vi "Cook Dinner.vi"() -> ()   [LabVIEW 2011]
uses:
  Chef/Chef.lvclass
  Microwave/Microwave.lvclass
  Toaster/Toaster.lvclass
  Oven/Oven.lvclass
panel:
  in  "Steam":bool
  in  "Toast":bool
  in  "Stop":bool
  in  "Broil":bool
  in  "Braise":bool
  in  "Bake":bool
  in  "Select Appliance":string(combo)="Oven"
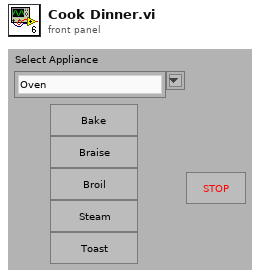
[diagram p1: front panel]
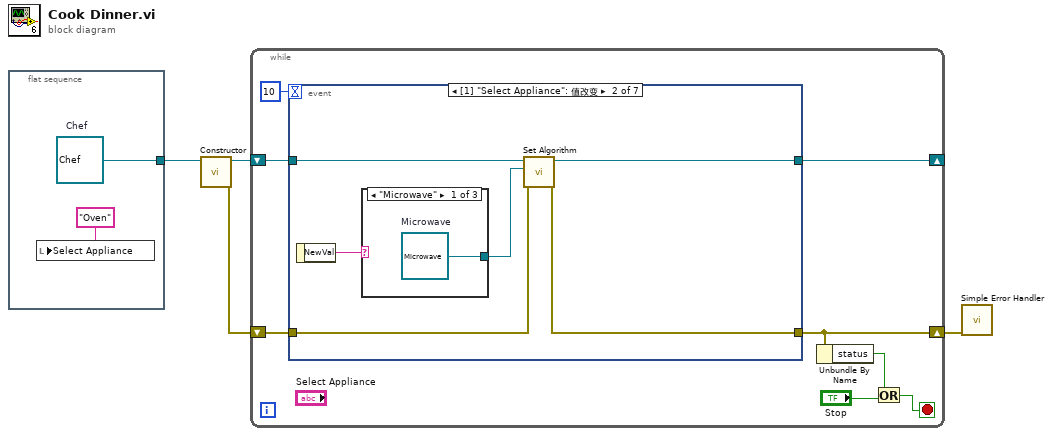
[diagram p0: block diagram]
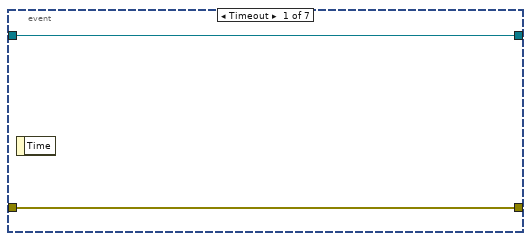
[diagram p2: hidden frame]
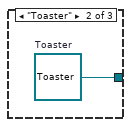
[diagram p3: hidden frame]
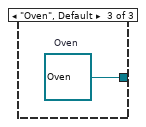
[diagram p4: hidden frame]
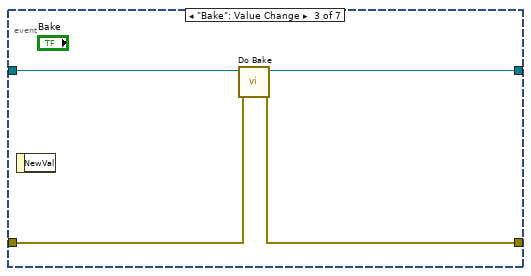
[diagram p5: hidden frame]
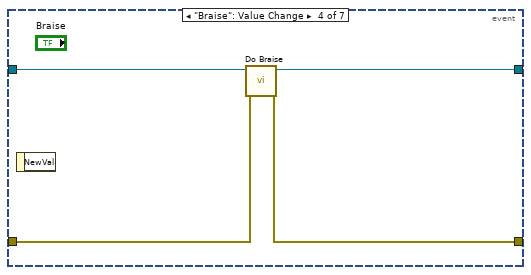
[diagram p6: hidden frame]
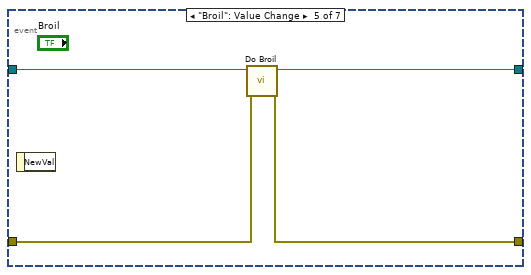
[diagram p7: hidden frame]
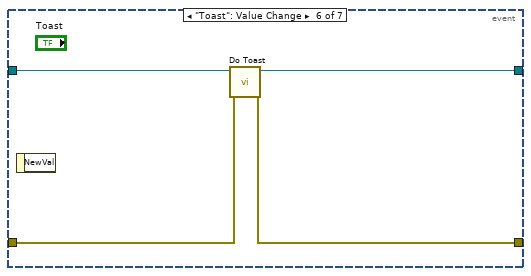
[diagram p8: hidden frame]
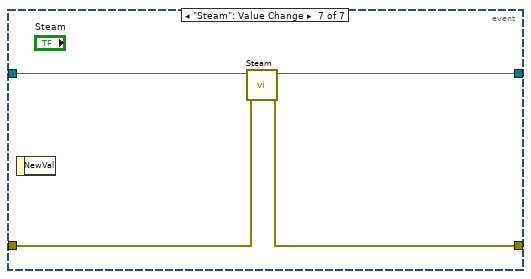
[diagram p9: hidden frame]
diagram:
  n1 = flat-sequence {
    tunnel: [w6] -> w4
    frame #0 {
      w6 = refnum<class "Chef.lvclass"> refnum  # Chef
      n2 = local write "Select Appliance"("Oven") -> ()
    }
  }
  n3 = call-dynamic "Constructor.vi"("Chef in"=w4) -> ("error out"=w2:errorcluster, "Chef out"=w3:refnum<class "Chef.lvclass">)  [unwired: 9 in]
  n4 = while {
    shift-right: [w12] -> _
    shift-left: w3 -> [w14]
    shift-right: [w11] -> w1
    shift-left: w2 -> [w13]
    stop <- w9 stop-if-true
    n5 = event shown="[1] \"Select Appliance\": 值改变" {
      selector: _ -> [_ _ _ _ _ _ _]
      dyn-events: _ -> [_ _ _ _ _ _ _]
      timeout: 10 -> [_ _ _ _ _ _ _]
      tunnel: w14 -> [w16 w22 w29 w33 w37 w41 w45]
      tunnel: [w15 w20 w26 w30 w34 w38 w42] -> w11
      tunnel: w13 -> [w15 w19 w27 w31 w35 w39 w43]
      tunnel: [w16 w18 w28 w32 w36 w40 w44] -> w12
      event Timeout {
        n6 = event-data() -> ()  [unwired: 1 in, 1 out]
      }
      event "Select Appliance": Value Change {
        n7 = event-data() -> ("NewVal"=w21:string)  [unwired: 1 in]
        n8 = case shown="\"Microwave\"" w21 {
          tunnel: [w23 w24 w25] -> w17
          frame "Microwave" {
            w23 = refnum<class "Microwave.lvclass"> refnum  # Microwave
          }
          frame "Toaster" {
            w24 = refnum<class "Toaster.lvclass"> refnum  # Toaster
          }
          frame "Oven", Default {
            w25 = refnum<class "Oven.lvclass"> refnum  # Oven
          }
        }
        n9 = call-dynamic "Set Algorithm.vi"("error in (no error)"=w19, "Appliance"=w17, "Chef in"=w22) -> ("error out"=w20:errorcluster, "Chef out"=w18:refnum<class "Chef.lvclass">)  [unwired: 7 in]
      }
      event "Bake": Value Change {
        n10 = event-data() -> ()  [unwired: 1 in, 1 out]
        n11 = call-dynamic "Do Bake.vi"("error in (no error)"=w27, "Chef in"=w29) -> ("error out"=w26:errorcluster, "Chef out"=w28:refnum<class "Chef.lvclass">)  [unwired: 8 in]
      }
      event "Braise": Value Change {
        n12 = event-data() -> ()  [unwired: 1 in, 1 out]
        n13 = call-dynamic "Do Braise.vi"("error in (no error)"=w31, "Chef in"=w33) -> ("error out"=w30:errorcluster, "Chef out"=w32:refnum<class "Chef.lvclass">)  [unwired: 8 in]
      }
      event "Broil": Value Change {
        n14 = event-data() -> ()  [unwired: 1 in, 1 out]
        n15 = call-dynamic "Do Broil.vi"("error in (no error)"=w35, "Chef in"=w37) -> ("error out"=w34:errorcluster, "Chef out"=w36:refnum<class "Chef.lvclass">)  [unwired: 8 in]
      }
      event "Toast": Value Change {
        n16 = event-data() -> ()  [unwired: 1 in, 1 out]
        n17 = call-dynamic "Do Toast.vi"("error in (no error)"=w39, "Chef in"=w41) -> ("error out"=w38:errorcluster, "Chef out"=w40:refnum<class "Chef.lvclass">)  [unwired: 8 in]
      }
      event "Steam": Value Change {
        n18 = event-data() -> ()  [unwired: 1 in, 1 out]
        n19 = call-dynamic "Steam.vi"("error in (no error)"=w43, "Chef in"=w45) -> ("error out"=w42:errorcluster, "Chef out"=w44:refnum<class "Chef.lvclass">)  [unwired: 8 in]
      }
    }
    n20 = Unbundle By Name(w11) -> ("status"=w8:bool)
    n21 = Or(x=w8, y="Stop") -> (x .or. y?=w9:bool)
  }
  n22 = call <vilib>:"Simple Error Handler.vi"("error in (no error)"=w1) -> ()  [unwired: 4 in, 5 out]
